vi "Calibrate.vi"(8 "error in (no error)":errorcluster, 11 "Santec in":refnum<class "Santec.lvclass">) -> (0 "error out":errorcluster, 3 "Santec out":refnum<class "Santec.lvclass">)   [LabVIEW 2014, in "Santec.lvclass"]
uses:
  Santec.lvclass
  Laser.lvclass
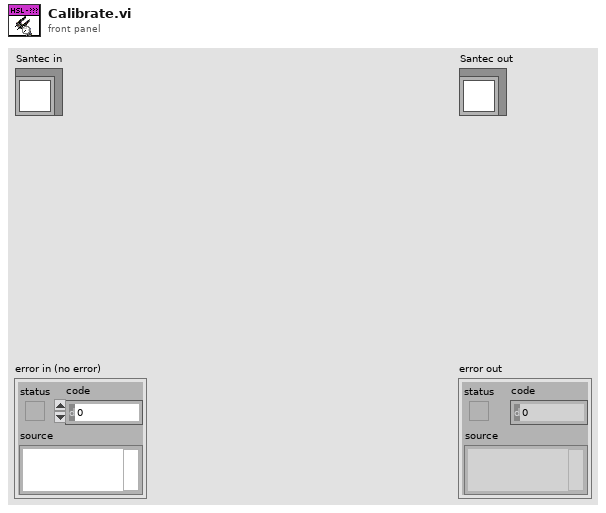
[diagram p1: front panel]
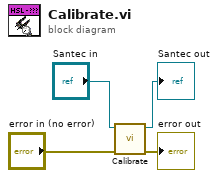
[diagram p0: block diagram]
diagram:
  n1 = call-parent "Calibrate.vi"("error in (no error)"="error in (no error)", "Laser in"="Santec in") -> ("error out"=→"error out":errorcluster, "Laser out"=→"Santec out":refnum<class "Santec.lvclass">)  [unwired: 8 in]
